vi "Update Image Table.vi"(8 "error in (no error)":errorcluster, 9 "Image Path":string, 10 "response":string, 11 "DB Path":string) -> (0 "error out":errorcluster)   [LabVIEW 2024]
uses:
  <vilib>/drjdpowell/SQLite Library/SQL Connection/Open (string).vi
  <vilib>/Analysis/baseanly.llb/Mean (DBL).vi
  <vilib>/drjdpowell/SQLite Library/SQL Connection/Execute SQL (No results).vi
  <vilib>/drjdpowell/SQLite Library/SQL Connection/Execute SQL.vi
  <vilib>/drjdpowell/SQLite Library/SQL Connection/Connection.lvclass
  <vilib>/drjdpowell/SQLite Library/SQLite.lvlib
  <vilib>/Analysis/NI_AALBase.lvlib
panel:
  out "Merged Boxes?":bool
  out "x2":dbl[](array[numeric])
  out "x1":dbl[](array[numeric])
  out "Column Names":string[](array[string])
  out "Feature Data":dbl[][](array[numeric])
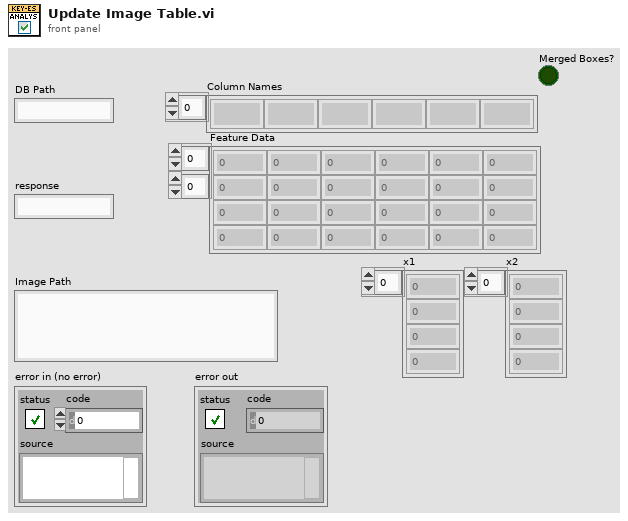
[diagram p1: front panel]
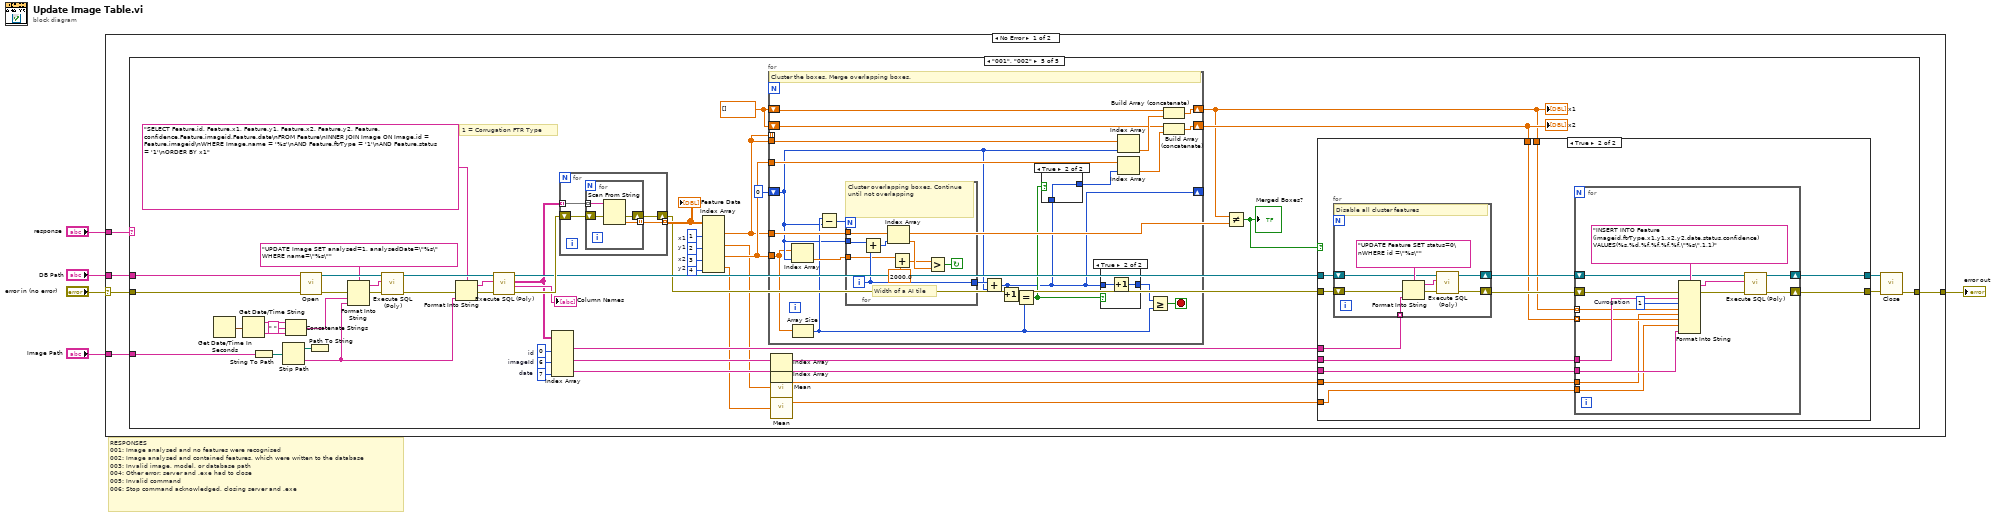
[diagram p0: block diagram]
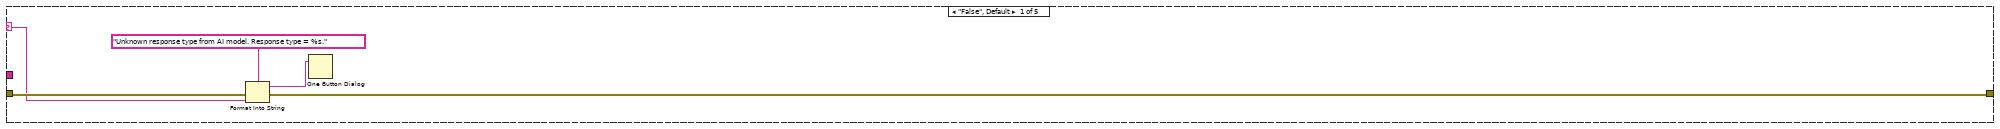
[diagram p2: hidden frame]
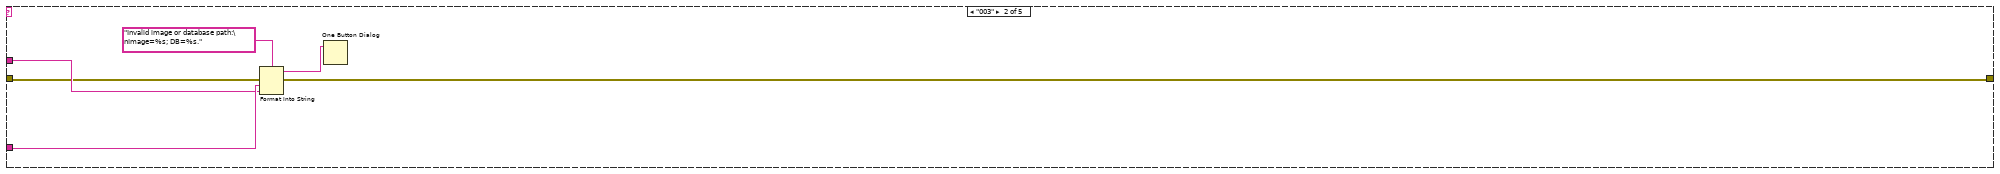
[diagram p3: hidden frame]
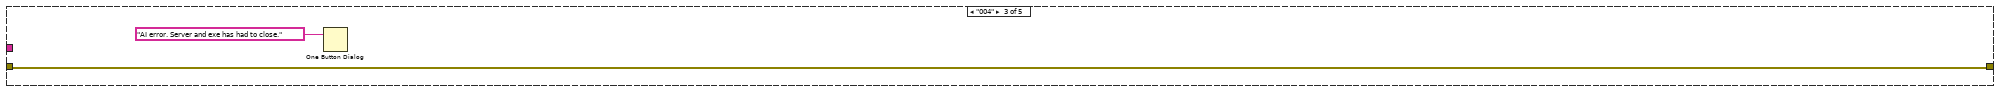
[diagram p4: hidden frame]
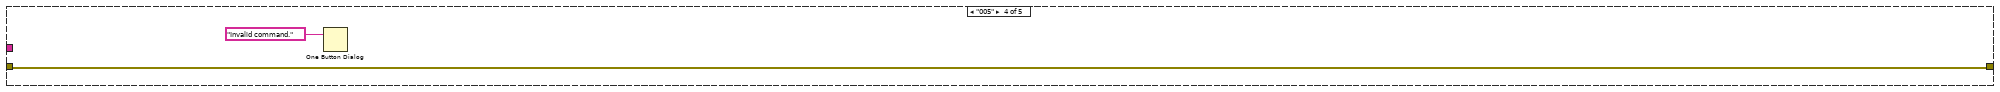
[diagram p5: hidden frame]
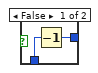
[diagram p8: hidden frame]
diagram:
  # "RESPONSES\n001: Image analysed and no features were recognised\n002: Image analysed and contained features, which were written to the database\n003: Invalid image, model, or database path\n004: Other error: server and .exe had to close\n005: Invalid command\n006: Stop command acknowledged, closing server and .exe"
  n1 = case shown="No Error" "error in (no error)" {
    selector: "error in (no error)" -> [w8 w160]
    tunnel: [w10 w160] -> w5
    tunnel: "DB Path" -> [w9 _]
    tunnel: "Image Path" -> [w7 _]
    tunnel: "response" -> [w6 _]
    frame No Error {
      n2 = case shown="\"001\", \"002\"" w6 {
        selector: w6 -> [w11 _ _ _ _]
        tunnel: [w12 w16 w23 w25 w73] -> w10
        tunnel: w9 -> [_ w19 _ _ w72]
        tunnel: w8 -> [w13 w18 w23 w25 w71]
        tunnel: w7 -> [_ w20 _ _ w68]
        frame "False", Default {
          n3 = Format Into String(format string="Unknown response type from AI model. Response type = %s." ("message"), error in=w13, w11) -> (resulting string=w14:string, error out=w12:errorcluster)  [unwired: 1 in]
          n4 = One Button Dialog(message=w14) -> ()  [unwired: 1 in, 1 out]
        }
        frame "003" {
          n5 = Format Into String(format string="Invalid image or database path:\nImage=%s; DB=%s." ("message"), error in=w18, w20, w19) -> (resulting string=w17:string, error out=w16:errorcluster)  [unwired: 1 in]
          n6 = One Button Dialog(message=w17) -> ()  [unwired: 1 in, 1 out]
        }
        frame "004" {
          n7 = One Button Dialog(message="AI error. Server and exe has had to close.") -> ()  [unwired: 1 in, 1 out]
        }
        frame "005" {
          n8 = One Button Dialog(message="Invalid command.") -> ()  [unwired: 1 in, 1 out]
        }
        frame "001", "002" {
          w36 = 7  # date
          w37 = 6  # imageId
          w39 = 0  # id
          w49 = dbl[] [] ("subarray")
          w50 = 4  # y2
          w51 = 3  # x2
          w52 = 2  # y1
          w53 = 1  # x1
          # "1 = Corrugation FTR Type"
          n9 = Get Date/Time In Seconds() -> (seconds since 1Jan1904=w63:timestamp)
          n10 = Get Date/Time String(seconds (now)=w63) -> (date string=w66:string, time string=w67:string)  [unwired: 2 in]
          n11 = String To Path(string=w68) -> (path=w69:path)
          n12 = Strip Path(path=w69) -> (stripped path=w70:path, name=w57:string)
          n13 = Concatenate Strings(w66, " " ("string"), w67) -> (w64:string)
          n14 = call-poly <vilib>:"Open.vi"("error in (no error)"=w71, "db file"=w72) -> ("error out"=w78:errorcluster, "SQLite Connection"=w76:refnum<class "Connection.lvclass">)  [unwired: 8 in]
          n15 = Path To String(path=w70) -> ()  [unwired: 1 out]
          n16 = Format Into String(format string="UPDATE Image SET analysed=1, analysedDate=\"%s\" WHERE name=\"%s\"", error in=w78, w64, w57) -> (resulting string=w75:string, error out=w77:errorcluster)  [unwired: 1 in]
          n17 = call-poly <vilib>:"Execute SQL (Poly).vi"("error in (no error)"=w77, "SQL"=w75, "SQLite Connection in"=w76) -> ("error out"=w59:errorcluster, "SQLite Connection"=w62:refnum<class "Connection.lvclass">)  [unwired: 7 in]
          n18 = Format Into String(format string="SELECT Feature.id, Feature.x1, Feature.y1, Feature.x2, Feature.y2, Feature.confidence,Feature.imageid,Feature.date\nFROM Feature\nINNER JOIN Image ON Image.id = Feature.imageid\nWHERE Image.name = '%s'\nAND Feature.ftrType = '1'\nAND Feature.status = '1'\nORDER BY x1", error in=w59, w57) -> (resulting string=w60:string, error out=w58:errorcluster)  [unwired: 1 in]
          n19 = call-poly <vilib>:"Execute SQL (Poly).vi"("error in (no error)"=w58, "SQL"=w60, "SQLite Connection in"=w62) -> ("error out"=w56:errorcluster, "Column Names"=→"Column Names":string[], "Result Set"=w40:string[][], "SQLite Connection"=w45:refnum<class "Connection.lvclass">)  [unwired: 5 in]
          n20 = Index Array(array=w40, index (col) #1=w39, index (col) #2=w37, index (col) #3=w36) -> (element #1=w38:string[], element #2=w35:string[], element #3=w34:string[])  [unwired: 3 in]
          n21 = for {
            tunnel: w40 -> [w155] mode=indexing
            tunnel: [w154] -> w54 mode=indexing
            shift-right: [w152] -> w44
            shift-left: w56 -> [w153]
            n22 = for {
              tunnel: w155 -> [w159] mode=indexing
              tunnel: [w158] -> w154 mode=indexing
              shift-right: [w156] -> w152
              shift-left: w153 -> [w157]
              n23 = Scan From String(input string=w159, error in=w157) -> (error out=w156:errorcluster, output 1=w158:dbl)  [unwired: 3 in, 2 out]
            }
          }
          "Feature Data" <- w54
          n24 = Index Array(array=w54, index (col) #1=w53, index (col) #2=w52, index (col) #3=w51, index (col) #4=w50) -> (element #1=w46:dbl[], element #2=w33:dbl[], element #3=w48:dbl[], element #4=w32:dbl[])  [unwired: 4 in]
          n25 = for {
            tunnel: w46 -> [w126]
            tunnel: w48 -> [w116]
            shift-right: [w133] -> w26
            shift-left: w49 -> [w135]
            shift-right: [w131] -> w27
            shift-left: w49 -> [w132]
            tunnel: w48 -> [w130]
            tunnel: w46 -> [w136]
            shift-right: [w118] -> _
            shift-left: 0 -> [w119]
            tunnel: w46 -> [_] mode=indexing
            stop <- w128 stop-if-true
            # "Cluster the boxes. Merge overlapping boxes."
            n26 = Index Array(array=w116, index=w119) -> (element=w125:dbl)
            n27 = Array Size(array=w116) -> (size(s)=w121:i32)
            n28 = Subtract(x=w121, y=w119) -> (x-y=w120:i32)
            n29 = for {
              N: w120 -> [_]
              tunnel: [w148] -> w127
              tunnel: w126 -> [w150]
              tunnel: w119 -> [w149]
              tunnel: w125 -> [w146]
              i -> [w148]
              stop <- w151 continue-if-true
              # "Width of a AI tile"
              # "Cluster overlapping boxes. Continue until not overlapping"
              n30 = Add(x=w149, y=w148) -> (x+y=w147:i32)
              n31 = Index Array(array=w150, index=w147) -> (element=w145:dbl)
              n32 = Add(x=w146, y=2000.0) -> (x+y=w144:dbl)
              n33 = Greater?(x=w144, y=w145) -> (0:w151:bool)
            }
            n34 = Add(x=w127, y=w119) -> (x+y=w118:i32)
            n35 = Increment(x=w118) -> (x+1=w117:i32)
            n36 = Equal?(x=w117, y=w121) -> (x = y?=w122:bool)
            n37 = case shown="True" w122 {
              tunnel: w118 -> [w141 w142]
              tunnel: [w140 w142] -> w124
              frame False {
                n38 = Decrement(x=w141) -> (x-1=w140:i32)
              }
              frame True {
              }
            }
            n39 = case shown="True" w122 {
              tunnel: w118 -> [w137 w139]
              tunnel: [w137 w138] -> w123
              frame False {
              }
              frame True {
                n40 = Increment(x=w139) -> (x+1=w138:i32)
              }
            }
            n41 = Index Array(array=w136, index=w119) -> (element=w134:dbl)
            n42 = Index Array(array=w130, index=w124) -> (element=w129:dbl)
            n43 = Greater Or Equal?(x=w123, y=w121) -> (x >= y?=w128:bool)
            n44 = Build Array (concatenate)(w135, w134) -> (w133:dbl[])
            n45 = Build Array (concatenate)(w132, w129) -> (w131:dbl[])
          }
          "x1" <- w26
          "x2" <- w27
          n46 = Index Array(array=w35) -> (element=w29:string)  [unwired: 1 in]
          n47 = Index Array(array=w34) -> (element=w28:string)  [unwired: 1 in]
          n48 = call-poly <vilib>:"Mean.vi"("X"=w33) -> ("mean"=w31:dbl)  [unwired: 1 out]
          n49 = call-poly <vilib>:"Mean.vi"("X"=w32) -> ("mean"=w30:dbl)  [unwired: 1 out]
          n50 = Not Equal?(x=w26, y=w46) -> (x != y?=w41:bool)
          "Merged Boxes?" <- w41
          n51 = case shown="True" w41 {
            tunnel: w45 -> [w80 w93]
            tunnel: w44 -> [w79 w92]
            tunnel: [w79 w87] -> w43
            tunnel: [w80 w88] -> w42
            tunnel: w38 -> [_ w91]
            tunnel: w29 -> [_ w86]
            tunnel: w28 -> [_ w85]
            tunnel: w31 -> [_ w84]
            tunnel: w30 -> [_ w83]
            tunnel: w27 -> [_ w82]
            tunnel: w26 -> [_ w81]
            frame False {
            }
            frame True {
              n52 = for {
                shift-right: [w109] -> w89
                shift-left: w93 -> [w112]
                shift-right: [w110] -> w90
                shift-left: w92 -> [w111]
                tunnel: w91 -> [w108] mode=indexing
                # "Disable all cluster features"
                n53 = Format Into String(format string="UPDATE Feature SET status=0\nWHERE id =\"%s\"", error in=w111, w108) -> (resulting string=w114:string, error out=w113:errorcluster)  [unwired: 1 in]
                n54 = call-poly <vilib>:"Execute SQL (Poly).vi"("error in (no error)"=w113, "SQL"=w114, "SQLite Connection in"=w112) -> ("error out"=w110:errorcluster, "SQLite Connection"=w109:refnum<class "Connection.lvclass">)  [unwired: 7 in]
              }
              n55 = for {
                shift-right: [w103] -> w87
                shift-left: w90 -> [w106]
                shift-right: [w104] -> w88
                shift-left: w89 -> [w105]
                tunnel: w86 -> [w101]
                tunnel: w85 -> [w100]
                tunnel: w84 -> [w96]
                tunnel: w83 -> [w95]
                tunnel: w82 -> [w97] mode=indexing
                tunnel: w81 -> [w98] mode=indexing
                w99 = 1  # Currogation
                n56 = Format Into String(format string="INSERT INTO Feature (imageid,ftrType,x1,y1,x2,y2,date,status,confidence) VALUES(%s,%d,%f,%f,%f,%f,\"%s\",1,1)", error in=w106, w101, w99, w98, w96, w97, w95, w100) -> (resulting string=w94:string, error out=w102:errorcluster)  [unwired: 1 in]
                n57 = call-poly <vilib>:"Execute SQL (Poly).vi"("error in (no error)"=w102, "SQL"=w94, "SQLite Connection in"=w105) -> ("error out"=w103:errorcluster, "SQLite Connection"=w104:refnum<class "Connection.lvclass">)  [unwired: 7 in]
              }
            }
          }
          n58 = call-dynamic "Close.vi"("error in (no error)"=w43, "SQLite Connection in"=w42) -> ("error out"=w73:errorcluster)  [unwired: 9 in]
        }
      }
    }
    frame Error {
    }
  }
  "error out" <- w5
